vi "Read Color.vi"(9 "Cluster in":refnum<class "Cluster.lvclass">) -> (3 "Cluster out":refnum<class "Cluster.lvclass">, 4 "Color":u32(colorbox))   [LabVIEW 2014, in "Cluster.lvclass"]
uses:
  Cluster.lvclass
  Cluster.lvclass/Cluster.ctl
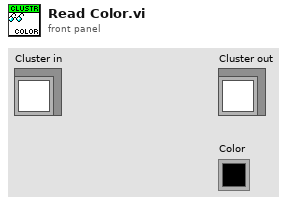
[diagram p1: front panel]
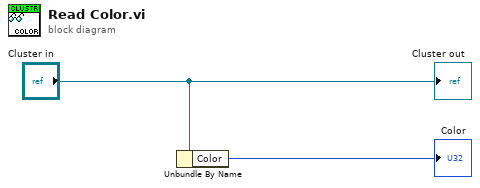
[diagram p0: block diagram]
diagram:
  n1 = Unbundle By Name("Cluster in") -> ("Color"=→"Color":u32)
  "Cluster out" <- "Cluster in"
